vi "MToolT8511.vi"(8 "error in (no error)":errorcluster, 10 "VISA resource name":refnum<visa-resource-name>="USB0::0x2A8D::0xB318::MY59430005::INSTR", 11 "ChangeStatus":u16(ring) items=["IT8511", "34450A", "WRBuff"]) -> (0 "error out":errorcluster, 3 "read buffer":string)   [LabVIEW 2019]
panel:
  out "Numeric":dbl
  out "μA":dbl format="%#_6f"
  out "hex integer string":string
  in  "Ringfor34450A":u16(ring) items=["SYSTem:VERSion?", "SYSTem:ERRor?", "*IDN?", "MEAS:CURR:DC?", "MEAS:VOLT?", "SYSTem:ERRor?"]
  in  "RingforIT8511":u16(ring) items=["SYSTem:VERSion?", "SYSTem:ERRor?", "*IDN?", "MEAS:CURR:DC?", "MEAS:VOLT?", "MEAS:VOLT:DC?"]
  in  "milliseconds to wait":u32
  in  "write buffer":string
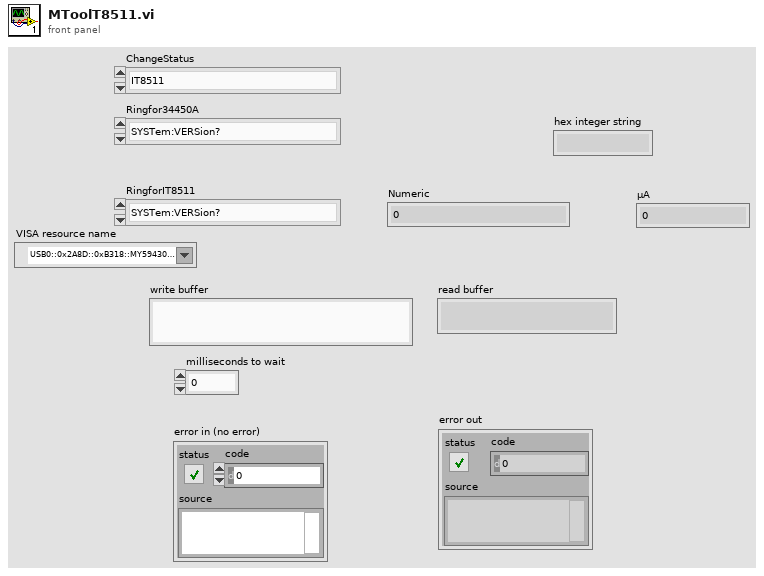
[diagram p1: front panel]
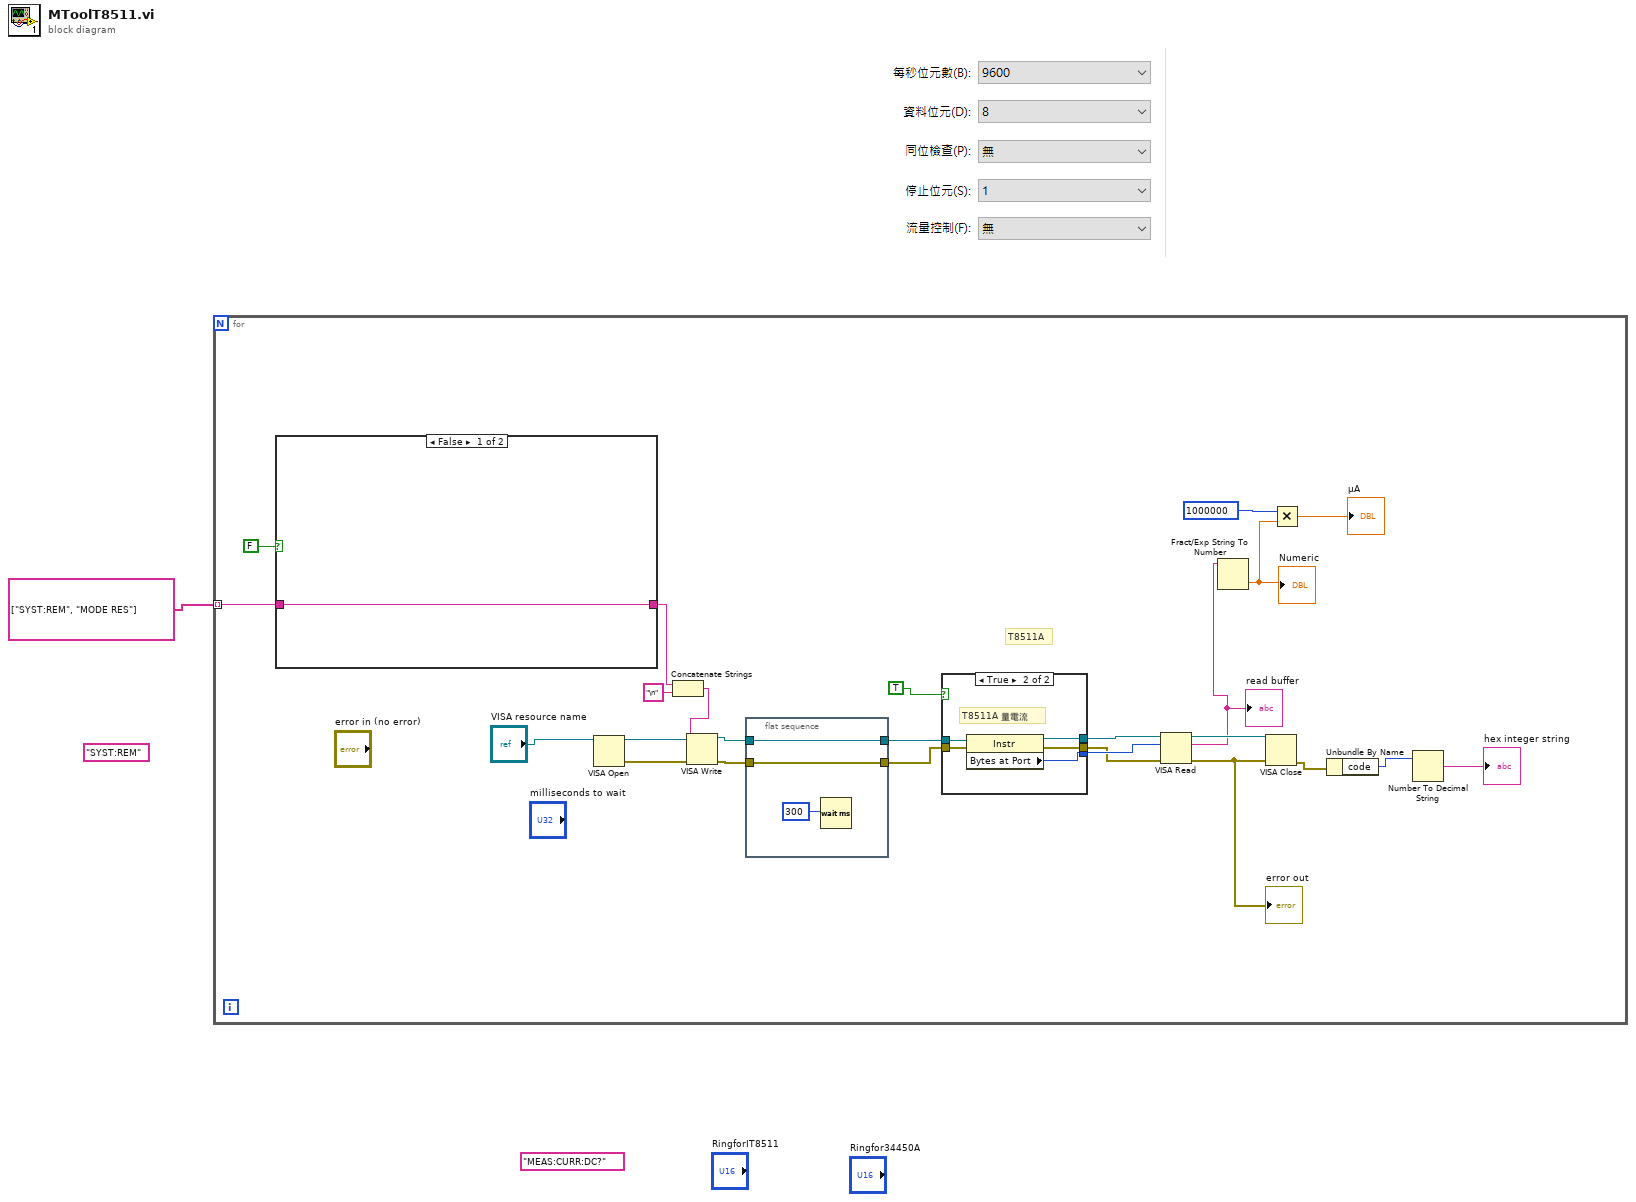
[diagram p0: block diagram]
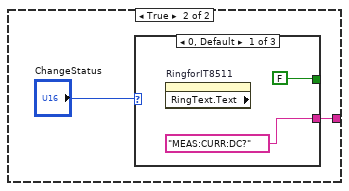
[diagram p2: hidden frame]
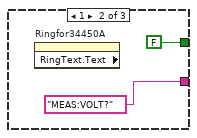
[diagram p3: hidden frame]
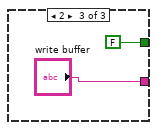
[diagram p4: hidden frame]
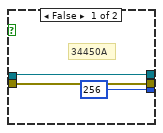
[diagram p5: hidden frame]
diagram:
  (unwired) "SYST:REM" ("string")
  (unwired) "MEAS:CURR:DC?" ("string")
  n1 = for {
    tunnel: string[] ["SYST:REM", "MODE RES"] -> [w2] mode=indexing
    # "T8511A"
    n2 = case shown="False" FALSE {
      tunnel: [w27 w28] -> w10
      tunnel: w2 -> [w27 _]
      frame False {
      }
      frame True {
        n3 = case shown="0, Default" "ChangeStatus" {
          tunnel: ["MEAS:CURR:DC?" ("string") "MEAS:VOLT?" ("string") "write buffer"] -> w28
          tunnel: [FALSE FALSE FALSE] -> _
          frame 0, Default {
            n4 = property on="RingforIT8511" class="Ring (strict)" props=["RingText", "Text"]() -> ()  [unwired: 2 in, 3 out]
          }
          frame 1 {
            n5 = property on="Ringfor34450A" class="Ring (strict)" props=["RingText", "Text"]() -> ()  [unwired: 2 in, 3 out]
          }
          frame 2 {
          }
        }
      }
    }
    n6 = VISA Open(VISA resource name="VISA resource name") -> (VISA resource name=w26:refnum<visa-resource-name>, error out=w25:errorcluster)  [unwired: 4 in]
    n7 = Concatenate Strings(w10, "\n" ("string")) -> (w15:string)
    n8 = VISA Write(VISA resource name=w26, write buffer=w15, error in (no error)=w25) -> (VISA resource name out=w20:refnum<visa-resource-name>, error out=w23:errorcluster)  [unwired: 1 out]
    n9 = flat-sequence {
      tunnel: w23 -> [w46]
      tunnel: [w46] -> w19
      tunnel: [w45] -> w21
      tunnel: w20 -> [w45]
      frame #0 {
        n10 = Wait (ms)(milliseconds to wait=300) -> ()  [unwired: 1 out]
      }
    }
    n11 = case shown="True" TRUE {
      tunnel: [u32 256 ("Bytes at Port") w43] -> w22
      tunnel: w21 -> [w38 w42]
      tunnel: w19 -> [w37 w41]
      tunnel: [w37 w40] -> w18
      tunnel: [w38 w39] -> w17
      frame False {
        # "34450A"
      }
      frame True {
        # "T8511A 量電流"
        n12 = property class="Instr"(reference=w42, error in=w41) -> (reference out=w39:refnum<visa-resource-name>, error out=w40:errorcluster, "Bytes at Port"=w43:u32)
      }
    }
    n13 = VISA Read(VISA resource name=w17, byte count=w22, error in (no error)=w18) -> (VISA resource name out=w24:refnum<visa-resource-name>, read buffer=w5:string, error out=w11:errorcluster)  [unwired: 1 out]
    "read buffer" <- w5
    "error out" <- w11
    n14 = Fract/Exp String To Number(string=w5) -> (number=w7:dbl)  [unwired: 3 in, 1 out]
    "Numeric" <- w7
    n15 = VISA Close(VISA resource name=w24, error in (no error)=w11) -> (error out=w12:errorcluster)
    n16 = Multiply(x=1000000, y=w7) -> (x*y=→"μA":dbl)
    n17 = Unbundle By Name(w12) -> ("code"=w14:i32)
    n18 = Number To Decimal String(number=w14) -> (decimal integer string=→"hex integer string":string)  [unwired: 1 in]
  }
